vi "Initialize.vi"(5 "components directory (default)":path, 7 "framework options":T1={"FIFO Options"={"Infinite Timeouts"=FALSE}, "Thread Options"={"Show FP On Call"=FALSE, "Close FP After Call"=FALSE, "Allow Debugging"=FALSE}, "Plugin Options"={"Default Components"=FALSE}, "Performance Options"={"Measure Period"=FALSE, "Measure Rx/Tx Duration"=FALSE}, "Data Server Options"={"Enable Data Server"=FALSE, "Period"=100}} {"Data Server Options"."Period" format="%d ms"}, 8 "error in (no error)":errorcluster, 10 "Framework Configuration":refnum<class "Framework Configuration.lvclass">, 11 "Framework in":refnum<class "Framework.lvclass">) -> (0 "error out":errorcluster, 3 "Framework out":refnum<class "Framework.lvclass">)   [LabVIEW 2019, in "DSF Core.lvlib" / "Framework.lvclass"]
uses:
  Framework.lvclass
  Framework Options.ctl
  Typedefs/DSF FIFO Options.ctl
  Thread/Thread Options.ctl
  Typedefs/DSF Plugin Options.ctl
  Typedefs/DSF Performance Options.ctl
  Data Server Options.ctl
  Configuration/Core/Framework/Framework Configuration.lvclass
  Framework States.ctl
  <vilib>/NI/Memory Manager/Classes/Pointer/Pointer.lvclass/Pointer.ctl
  Framework Status/Framework Status.lvclass/Framework Status.ctl
  Performance/Performance.lvclass/Performance.ctl
  Pointers/Error/Error Pointer.lvclass/Error Pointer.ctl
  Framework.lvclass/Framework.ctl
  Thread/Thread.lvclass/Thread.ctl
  Interface/Interface.lvclass/Interface.ctl
  Thread/Logging/Logging Thread.lvclass/Logging Thread.ctl
  Buffers/Buffers.lvclass/Buffers.ctl
  Buffer/Buffer.lvclass/Buffer.ctl
  Transfer/Transfer.lvclass/Transfer.ctl
  Timing/Timing.lvclass/Timing.ctl
  Transfer Group/Transfer Group.lvclass/Transfer Group.ctl
  Component Loader/Component Loader.lvclass/Component Loader.ctl
  Component/Component.lvclass/Component.ctl
  Plugin/Plugin.lvclass/Plugin.ctl
  Thread/Plugin/Plugin Thread.lvclass/Plugin Thread.ctl
  Thread/Dispatcher/Dispatcher Thread.lvclass/Dispatcher Thread.ctl
  Thread/Data Server/Data Server Thread.lvclass/Data Server Thread.ctl
  Thread Manager/Thread Manager.lvclass/Thread Manager.ctl
  Component Loader/Load Components.vi
  Transfer Group/Subset Transfer Groups.vi
  Component Loader/Create.vi
  Plugin/Sort by Priority.vi
  Separate Inline and Async Plugins.vi
  Create Groups.vi
  Thread/Dispatcher/New.vi
  Performance/Create.vi
  Framework Status/Create Framework Status.vi
  <vilib>/NI/Memory Manager/Classes/Pointer/Allocate.vi
  <vilib>/NI/Memory Manager/Classes/Pointer/Write.vi
  <vilib>/NI/Memory Manager/Classes/Pointer/Write U8.vi
  Pointers/Error/New Error Pointer.vi
  Thread Manager/Launch All.vi
  Thread Manager/Create.vi
  Thread Manager/Run All.vi
  Thread/Logging/New Logging Thread.vi
  Plugin/Get Name.vi
  Plugin/Get Thread Interfaces.vi
  Interface/Logging/Send.vi
  Interface/Logging/Send Logging Command.vi
  Read State.vi
  Pointers/Error/Write Error Pointer.vi
  <vilib>/NI/Memory Manager/Classes/Pointer/Get Address.vi
  Thread/Data Server/Create Data Server Thread.vi
  Transfer Group/Sort Groups by ID.vi
  Plugin/Get Async Rx Transfer Groups.vi
  Plugin/Get Async Tx Transfer Groups.vi
  Plugin/Get Inline Rx Transfer Groups.vi
  Plugin/Get Inline Tx Transfer Groups.vi
  Transfer Group/Get Buffers.vi
  Transfer Group/Get Transfers.vi
  Transfer Group/Get Status.vi
  Plugin/Get Status.vi
  Get Status.vi
  Framework Status/Get Status Pointer.vi
  Timing/Create Timing (cluster).vi
  Plugin/Initialize Transfer Groups.vi
  Plugin/Initialize Threads.vi
  Framework Status/Get Plugin Pointers.vi
  Component Loader/Load Packed Library.vi
  Internal Components.vi
  Component/Get Name.vi
  Component Loader/Errors.vi
  Component Loader/Component Directory Not Found.vi
  Plugin/Get Timing.vi
  Timing/Is Inline.vi
  Plugin/Set Active.vi
  Transfer Group/Create Transfer Group.vi
  Interface/Dispatcher/New.vi
  Thread/Set Thread Parameters.vi
  Thread/Set Name.vi
  Thread/Dispatcher/Initialize Plugin Settings.vi
  Timing Status/Create.vi
  Timing Status/Write Timing Status.vi
  Status/Create.vi
  <vilib>/NI/Memory Manager/Classes/Pointer/Set Address.vi
  <vilib>/NI/Memory Manager/Classes/Pointer/Set Size.vi
  <vilib>/NI/Memory Manager/Classes/Pointer/Set Internal.vi
  <vilib>/NI/Memory Manager/Classes/Pointer/Write (No Check).vi
  <vilib>/NI/Memory Manager/Classes/Pointer/Write (No Check) U8.vi
  <vilib>/NI/Memory Manager/Classes/Pointer/Check Move.vi
  Pointers/Error/Error Size.vi
  Thread/Launch.vi
  Thread/Override State Pointer.vi
  <vilib>/NI/Memory Manager/Classes/Pointer/Subset.vi
  Thread/Override Error Pointer.vi
  Pointers/Error/Get Power Of 2.vi
  Thread/Run Thread.vi
  Interface/Logging/Create.vi
  Thread/Logging/Create Log File.vi
  Interface/Send Command.vi
  Interface/Errors.vi
  Interface/Dispatcher/Command Timeout.vi
  <vilib>/NI/Memory Manager/Classes/Pointer/Read.vi
  <vilib>/NI/Memory Manager/Classes/Pointer/Read U8.vi
  <vilib>/NI/Memory Manager/Classes/Pointer/Write 1D U8.vi
  <vilib>/NI/Memory Manager/Classes/Pointer/Clear.vi
  Interface/Plugin/Create.vi
  Transfer Group/Get ID.vi
  Timing/Create Timing.vi
  Transfer Group/Set Inline.vi
  Transfer Group/Initialize Status.vi
  Transfer Group/Set ID.vi
  Plugin/Configure Transfer Groups.vi
  Transceiver/New.vi
  Thread/Plugin/Initialize Transfer Groups.vi
  Thread/Plugin/Find.vi
  Status/Subset Status.vi
  Framework Status/Get Plugin Subset.vi
  Component Loader/Find Packed Library.vi
  Component Loader/Load Classes.vi
  Component Loader/Find Packed Library Classes.vi
  Component Configuration/Find.vi
  Component User Interface/Find.vi
  Component/Default Buffer Converter/Create.vi
  Component Loader/New Component Loader Error.vi
  <vilib>/NI/Memory Manager/VIs/Write String to Source.vi
  Transfer/Set Inline.vi
  Transfer/Initialize Transfer.vi
  Buffers/Subset Buffers.vi
  Transfer Group/Initialize Transfer Group.vi
  Interface/New Interface.vi
  Transfer Group/Get Thread.vi
  Timing Status/Timing Status Size.vi
  <vilib>/NI/Memory Manager/Classes/Pointer/Check Size.vi
  <vilib>/NI/Memory Manager/Classes/Pointer/Check Null Pointer.vi
  Status/Status Size.vi
  Status/Write Status 1D.vi
  <vilib>/NI/Memory Manager/Classes/Pointer/Check Count.vi
  <vilib>/NI/Memory Manager/Classes/Pointer/Check Bounds (Power of 2).vi
  <vilib>/NI/Memory Manager/Classes/Pointer/Is Null.vi
  <vilib>/NI/Memory Manager/Classes/Pointer/Deallocate.vi
  <vilib>/NI/Memory Manager/Classes/Pointer/Encapsulate.vi
  <vilib>/NI/Memory Manager/Classes/Pointer/Check Length.vi
  Thread/Read State.vi
  Thread/Write Command FIFO.vi
  Interface/Write RT FIFO.vi
  Interface/New Interface Error.vi
  <vilib>/NI/Memory Manager/Classes/Pointer/Read (No Check).vi
  <vilib>/NI/Memory Manager/Classes/Pointer/Read (No Check) U8.vi
  <vilib>/NI/Memory Manager/Classes/Pointer/Write (No Check) 1D U8.vi
  <vilib>/NI/Memory Manager/Classes/Pointer/Clear (No Check).vi
  Timing/Set Decimation.vi
  Timing/Set Offset.vi
  Timing/Set Priority.vi
  Timing/Errors.vi
  Timing/Invalid Offset.vi
  Timing/Invalid Priority.vi
  Transfer Group/Sort by Priority.vi
  Transfer Group/Separate Rx and Tx.vi
  Transfer Group/Separate Inline and Async.vi
  Timing/Get Priority.vi
  Plugin/Get ID.vi
  Thread/Set ID.vi
  <vilib>/Utility/error.llb/Clear Errors.vi
  Component/Get Objects.vi
  Component Loader/Find Packed Libraries.vi
  Component Loader/Component Not Found.vi
  Component Loader/Load Class.vi
  <vilib>/NI/Memory Manager/VIs/New Error Cluster.vi
  <vilib>/NI/Memory Manager/VIs/New Error Cluster (512B).vi
  Component Loader/Component Loader Error Info.vi
  <vilib>/NI/Memory Manager/VIs/Set Error Code.vi
  <vilib>/NI/Memory Manager/VIs/Set Error Status.vi
  <vilib>/NI/Memory Manager/VIs/Set Error Source.vi
  VIs/Constants/Constants.vi
  VIs/Constants/Engine Library Name.vi
  Transfer/Create Transfer.vi
  Buffer/Subset Buffer.vi
  Buffer/Set Buffer Size.vi
  Buffers/Create.vi
  Transfer Group/Create Return FIFO.vi
  Interface/Create RT FIFO.vi
  <vilib>/NI/Memory Manager/Classes/Pointer/Errors.vi
  <vilib>/NI/Memory Manager/Classes/Pointer/Out of Bounds.vi
  <vilib>/NI/Memory Manager/Classes/Pointer/Get Size.vi
  <vilib>/NI/Memory Manager/Classes/Pointer/Null Pointer.vi
  <vilib>/NI/Memory Manager/Classes/Pointer/Check Bounds.vi
  <vilib>/NI/Memory Manager/Classes/Pointer/Get Internal.vi
  <vilib>/NI/Memory Manager/Classes/Pointer/Zone.vi
  <vilib>/NI/Memory Manager/Classes/Pointer/Check Bounds (Pointer).vi
  Interface/Interface Error Info.vi
  Timing/New Timing Error.vi
  <vilib>/NI/Memory Manager/VIs/Write Numeric to Source.vi
  <vilib>/NI/Memory Manager/VIs/Write Numeric Scalar to Source (Base10 U64).vi
  Timing/Get Decimation.vi
  Transfer Group/Get Direction.vi
  Transfer Group/Get Timing.vi
  Transfer Group/Set Active.vi
  Component Loader/Class Not Found.vi
  Component Loader/Base Error Offset.vi
  VIs/Constants/Base Error Code.vi
  Buffer/Set Buffer Offset.vi
  <vilib>/NI/Memory Manager/Classes/Pointer/Write Pointer Size to Error.vi
  <vilib>/NI/Memory Manager/Classes/Pointer/Create Error.vi
  <vilib>/NI/Memory Manager/Classes/Pointer/Check Bounds (Buffer).vi
  Interface/Interface Error Offset.vi
  Timing/Timing Error Info.vi
  <vilib>/NI/Memory Manager/Constants/Constants.vi
  <vilib>/NI/Memory Manager/Constants/Library Name.vi
  <vilib>/NI/Memory Manager/Classes/Pointer/Pointer Error Info.vi
  <vilib>/NI/Memory Manager/Constants/Pointer Class Name.vi
  <vilib>/NI/Memory Manager/Classes/Pointer/Buffer Underflow.vi
  Timing/Base Error Offset.vi
  Status/Status Pointer.lvclass
  C:/Program Files (x86)/National Instruments/LabVIEW 2019/vi.lib/NI/Memory Manager/Classes/Pointer/Pointer.lvclass
  Timing Status/Timing Status Pointer.lvclass
  Pointers/Error/Error Pointer.lvclass
  Thread/Logging/Logging Thread.lvclass
  C:/Dev/GitHub/niveristand-data-sharing-framework-custom-device/Core/Classes/Thread/Thread.lvclass
  Interface/Logging/Logging Interface.lvclass
  C:/Dev/GitHub/niveristand-data-sharing-framework-custom-device/Core/Classes/Interface/Interface.lvclass
  Buffer/Buffer.lvclass
  Component/Default Buffer Converter/Default Buffer Converter Component.lvclass
  C:/Dev/GitHub/niveristand-data-sharing-framework-custom-device/Core/Classes/Component/Component.lvclass
  Thread/Plugin/Transceiver/Transceiver Thread.lvclass
  C:/Dev/GitHub/niveristand-data-sharing-framework-custom-device/Core/Classes/Thread/Plugin/Plugin Thread.lvclass
  Thread/Plugin/Plugin Thread.lvclass
  Interface/Plugin/Plugin Interface.lvclass
  Thread/Dispatcher/Dispatcher Thread.lvclass
  Interface/Dispatcher/Dispatcher Interface.lvclass
  Thread/Data Server/Data Server Thread.lvclass
  Configuration/Core/Framework/Get Plugin Configurations.vi
  Configuration/Core/Plugin/Get Thread Configurations.vi
  Configuration/Core/Thread/Get Group Configurations.vi
  Configuration/Core/Group/Get Core.vi
  Configuration/Core/Group/Get Transfer Configurations.vi
  Configuration/Core/Transfer/Get Name.vi
  <vilib>/Utility/libraryn.llb/Check if File or Folder Exists.vi
  Configuration/Core/Plugin/Get Components.vi
  <vilib>/Utility/libraryn.llb/Recursive File List.vi
  <vilib>/Utility/LVLibp/Get Exported File List.vi
  <vilib>/Utility/LVClass/Get LV Class Default Value.vi
  Configuration/Core/Plugin/Get Configuration.vi
  Configuration/Core/Thread/Get Core Configuration.vi
  Thread/Top.vi
  VIs/VI Name.vi
  Framework Status/Framework Status.lvclass
  Performance/Performance.lvclass
  <vilib>/NI/Memory Manager/Classes/Pointer/Pointer.lvclass
  Transfer Group/Transfer Group.lvclass
  Buffers/Buffers.lvclass
  Transfer/Transfer.lvclass
  Timing/Timing.lvclass
  Component Loader/Component Loader.lvclass
  Components/Buffer Converters/DSF Type Converter/Default Buffer Converter.lvclass
  Components/Buffer Converters/DSF Type Converter/User Interfaces/Default Buffer Converter User Interfaces.lvclass
  Components/Buffer Converters/DSF Type Converter/Configurations/Default Buffer Converter Configurations.lvclass
  Component User Interface/Component User Interfaces.lvclass
  Component Configuration/Component Configurations.lvclass
  Component/Component.lvclass
  Plugin/Plugin.lvclass
  Thread Manager/Thread Manager.lvclass
  Thread/Thread.lvclass
  Configuration/Core/Plugin/Plugin Configuration.lvclass
  Configuration/Core/Transfer/Transfer Configuration.lvclass
  Configuration/Core/Thread/Thread Configuration.lvclass
  DSF Core.lvlib
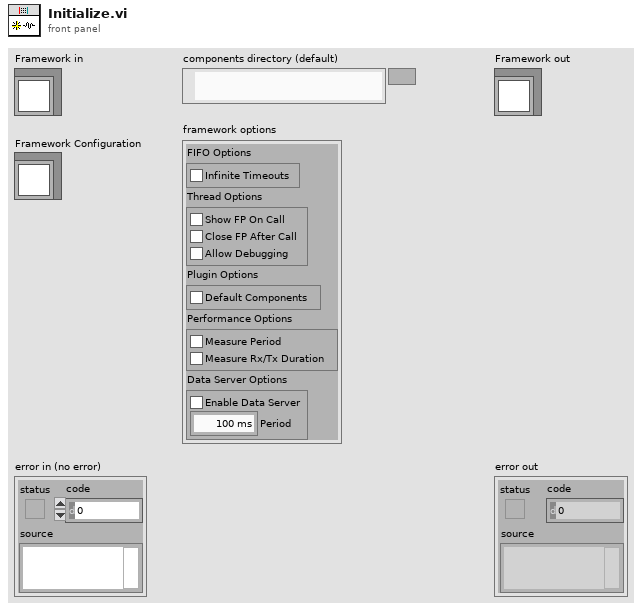
[diagram p1: front panel]
types:
  T1 = typedef "DSF Core.lvlib/Framework.lvclass/Framework Options.ctl" = cluster{"FIFO Options":T2, "Thread Options":T3, "Plugin Options":T4, "Performance Options":T5, "Data Server Options":T6}
  T2 = typedef "DSF Core.lvlib/Framework.lvclass/DSF FIFO Options.ctl" = cluster{"Infinite Timeouts":bool}
  T3 = typedef "DSF Core.lvlib/Thread.lvclass/Thread Options.ctl" = cluster{"Show FP On Call":bool, "Close FP After Call":bool, "Allow Debugging":bool}
  T4 = typedef "DSF Core.lvlib/Framework.lvclass/DSF Plugin Options.ctl" = cluster{"Default Components":bool}
  T5 = typedef "DSF Core.lvlib/DSF Performance Options.ctl" = cluster{"Measure Period":bool, "Measure Rx/Tx Duration":bool}
  T6 = typedef "DSF Core.lvlib/Framework.lvclass/Data Server Options.ctl" = cluster{"Enable Data Server":bool, "Period":u32}
  T7 = typedef "DSF Core.lvlib/Framework.lvclass/Framework States.ctl" = enum8{"Uninitialized", "Initialized", "Start", "Rx", "Tx", "Shutdown"}
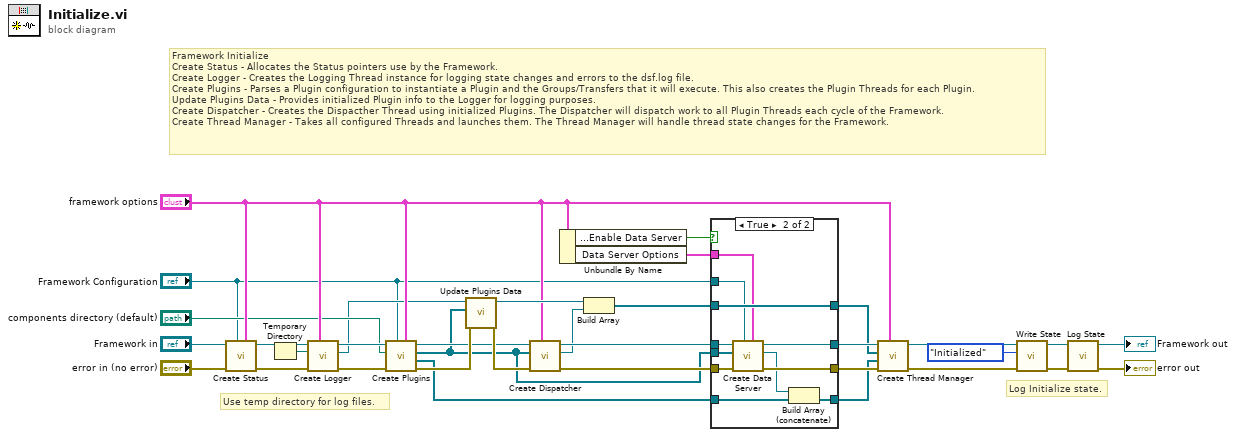
[diagram p0: block diagram]
diagram:
  # "Log Initialize state."
  # "Framework Initialize\nCreate Status - Allocates the Status pointers use by the Framework.\nCreate Logger - Creates the Logging Thread instance for logging state changes and errors to the dsf.log file.\nCreate Plugins - Parses a Plugin configuration to instantiate a Plugin and the Groups/Transfers that it will execute. This also creates the Plugin Threads for each Plugin.\nUpdate Plugins Data - Provides initialized Plugin info to the Logger for logging purposes.\nCreate Dispatcher - Creates the Dispacther Thread using initialized Plugins. The Dispatcher will dispatch work to all Plugin Threads each cycle of the Framework.\nCreate Thread Manager - Takes all configured Threads and launches them. The Thread Manager will handle thread state changes for the Framework."
  # "Use temp directory for log files."
  n1 = call "Create Status.vi"("framework options"="framework options", "Framework Configuration"="Framework Configuration", "error in (no error)"="error in (no error)", "Framework in"="Framework in") -> ("error out"=w29:errorcluster, "Framework out"=w30:refnum<class "Framework.lvclass">)  [unwired: 6 in]
  n2 = Temporary Directory() -> (w26:path)
  n3 = call "Create Logger.vi"("framework options"="framework options", "error in (no error)"=w29, "log file directory"=w26, "Framework in"=w30) -> ("error out"=w27:errorcluster, "Logging Thread"=w3:refnum<class "Logging Thread.lvclass">, "Framework out"=w28:refnum<class "Framework.lvclass">)  [unwired: 4 in, 1 out]
  n4 = call "Create Plugins.vi"("framework options"="framework options", "Framework Configuration"="Framework Configuration", "error in (no error)"=w27, "components directory"="components directory (default)", "Framework in"=w28) -> ("error out"=w33:errorcluster, "Plugin Threads"=w6:refnum<class "Plugin Thread.lvclass">[], "Plugins"=w17:refnum<class "Plugin.lvclass">[], "Framework out"=w32:refnum<class "Framework.lvclass">)  [unwired: 3 in]
  n5 = call "Update Plugins Data.vi"("error in (no error)"=w33, "Plugins"=w17, "Logging Thread in"=w3) -> ("error out"=w34:errorcluster, "Logging Thread out"=w12:refnum<class "Logging Thread.lvclass">)  [unwired: 7 in]
  n6 = call "Create Dispatcher.vi"("framework options"="framework options", "error in (no error)"=w34, "Plugins"=w17, "Framework in"=w32) -> ("error out"=w18:errorcluster, "Dispatcher Thread"=w11:refnum<class "Dispatcher Thread.lvclass">, "Framework out"=w16:refnum<class "Framework.lvclass">)  [unwired: 5 in]
  n7 = Unbundle By Name("framework options") -> ("Data Server Options.Enable Data Server"=w7:bool, "Data Server Options"=w8:T6)
  n8 = Build Array(w12, w11) -> (w10:refnum<class "Thread.lvclass">[])
  n9 = case shown="True" w7 {
    tunnel: w18 -> [w36 w49]
    tunnel: w17 -> [_ w48]
    tunnel: w16 -> [w37 w47]
    tunnel: [w37 w46] -> w15
    tunnel: [w38 w44] -> w14
    tunnel: [w36 w45] -> w13
    tunnel: w10 -> [w38 w44]
    tunnel: w8 -> [_ w40]
    tunnel: w6 -> [w35 w41]
    tunnel: [w35 w43] -> w5
    tunnel: "Framework Configuration" -> [_ w39]
    frame False {
    }
    frame True {
      n10 = call "Create Data Server.vi"("data server options"=w40, "Framework Configuration"=w39, "error in (no error)"=w49, "Plugins"=w48, "Framework in"=w47) -> ("error out"=w45:errorcluster, "Data Server Thread"=w42:refnum<class "Data Server Thread.lvclass">, "Framework out"=w46:refnum<class "Framework.lvclass">)  [unwired: 4 in]
      n11 = Build Array (concatenate)(w42, w41) -> (w43:refnum<class "Thread.lvclass">[])
    }
  }
  n12 = call "Create Thread Manager.vi"("framework options"="framework options", "error in (no error)"=w13, "Public Threads"=w5, "Private Threads"=w14, "Framework in"=w15) -> ("error out"=w24:errorcluster, "Framework out"=w25:refnum<class "Framework.lvclass">)  [unwired: 5 in]
  n13 = call "Write State.vi"("error in (no error)"=w24, "state"=Framework_States."Initialized", "Framework in"=w25) -> ("error out"=w21:errorcluster, "Framework out"=w22:refnum<class "Framework.lvclass">)  [unwired: 7 in]
  n14 = call "Log State.vi"("error in (no error)"=w21, "Framework in"=w22) -> ("error out"=→"error out":errorcluster, "Framework out"=→"Framework out":refnum<class "Framework.lvclass">)  [unwired: 8 in]
